vi "Connecting Points.vi"(1 "Boolean":bool, 3 "数组":dbl[][](array[numeric])) -> (0 "输出数组":T1(array[cluster]))   [LabVIEW 2016]
panel:
  out "输出数组 2":dbl[](array[numeric])
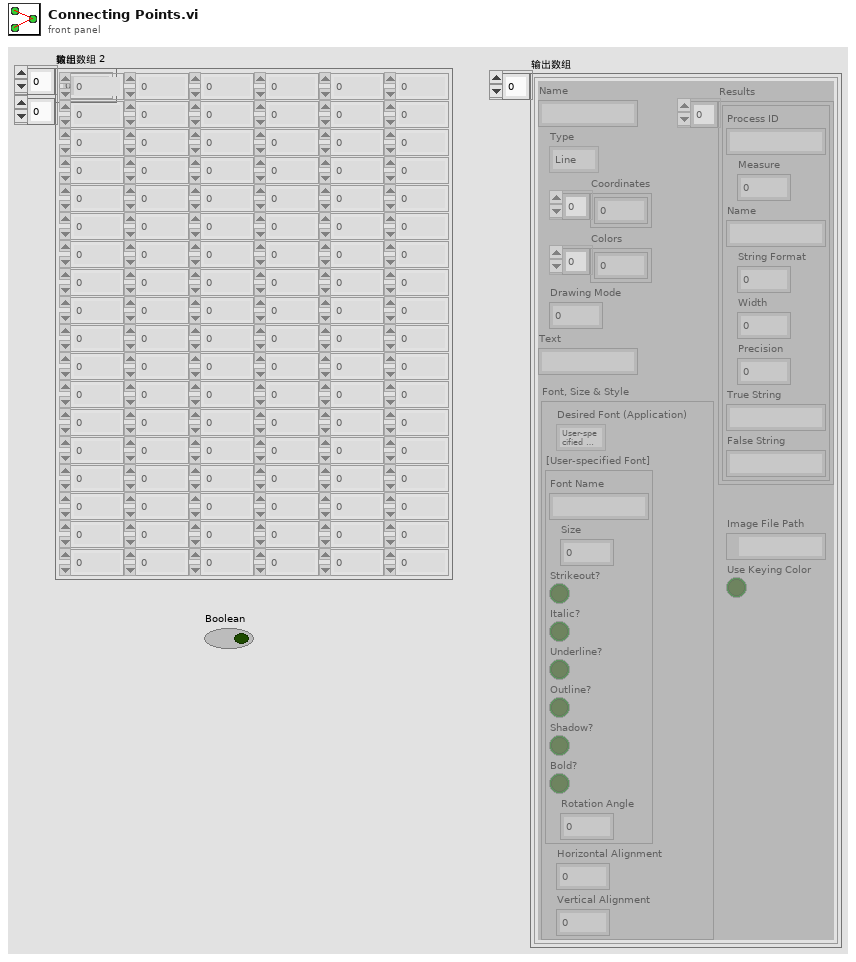
[diagram p1: front panel]
types:
  T1 = cluster{"Name":string, "Type":enum16{"Line", "Broken Line", "Free Hand Line", "Rotated Rectangle", "Oval", "Polygon", "Free Hand", "Bitmap", "Text"}, "Coordinates":i32[], "Colors":u32[], "Drawing Mode":u32, "Text":string, "Results":cluster{"Process ID":string, "Measure":u16, "Name":string, "String Format":u16, "Width":i16, "Precision":i16, "True String":string, "False String":string}[], "Font, Size & Style":cluster{"Desired Font (Application)":enum16{"User-specified Font", "Application Font", "System Font", "Dialog Font"}, "[User-specified Font]":cluster{"Font Name":string, "Size":i16, "Strikeout?":bool, "Italic?":bool, "Underline?":bool, "Outline?":bool, "Shadow?":bool, "Bold?":bool, "Rotation Angle":dbl}, "Horizontal Alignment":i16, "Vertical Alignment":i16}, "Image File Path":path, "Use Keying Color":bool}[]
  T2 = enum16{"Line", "Broken Line", "Free Hand Line", "Rotated Rectangle", "Oval", "Polygon", "Free Hand", "Bitmap", "Text"}
  T3 = cluster{"Name":string, "Type":enum16{"Line", "Broken Line", "Free Hand Line", "Rotated Rectangle", "Oval", "Polygon", "Free Hand", "Bitmap", "Text"}, "Coordinates":i32[], "Colors":u32[], "Drawing Mode":u32, "Text":string, "Results":cluster{"Process ID":string, "Measure":u16, "Name":string, "String Format":u16, "Width":i16, "Precision":i16, "True String":string, "False String":string}[], "Font, Size & Style":cluster{"Desired Font (Application)":enum16{"User-specified Font", "Application Font", "System Font", "Dialog Font"}, "[User-specified Font]":cluster{"Font Name":string, "Size":i16, "Strikeout?":bool, "Italic?":bool, "Underline?":bool, "Outline?":bool, "Shadow?":bool, "Bold?":bool, "Rotation Angle":dbl}, "Horizontal Alignment":i16, "Vertical Alignment":i16}, "Image File Path":path, "Use Keying Color":bool}
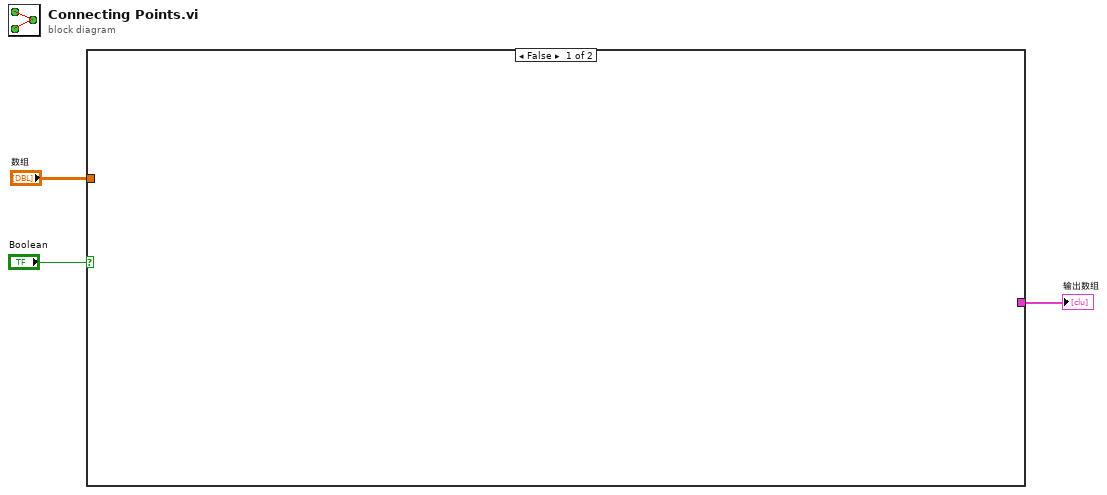
[diagram p0: block diagram]
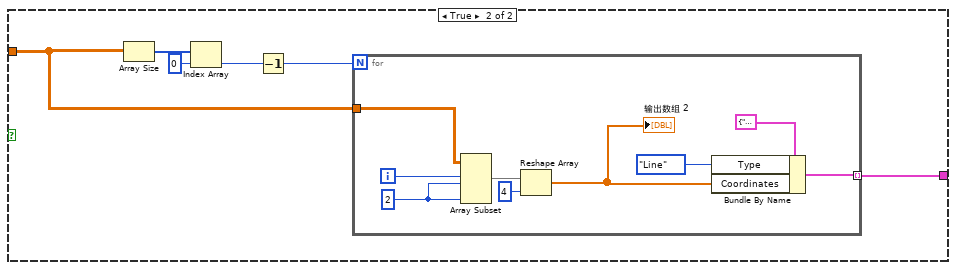
[diagram p2: hidden frame]
diagram:
  n1 = case shown="False" "Boolean" {
    tunnel: [_ w7] -> w3
    tunnel: "数组" -> [_ w6]
    frame False {
    }
    frame True {
      n2 = Array Size(array=w6) -> (size(s)=w8:i32[])
      n3 = Index Array(array=w8, index=0 ("索引")) -> (element=w5:i32)
      n4 = Decrement(x=w5) -> (x-1=w4:i32)
      n5 = for {
        N: w4 -> [_]
        tunnel: [w18] -> w7 mode=indexing
        tunnel: w6 -> [w15]
        i -> [w14]
        w13 = 2 ("长度")
        n6 = Array Subset(array=w15, index (row)=w14, length (row)=w13, length (col)=w13) -> (w12:dbl[][])  [unwired: 1 in]
        n7 = Reshape Array(w12, 4 ("维数大小")) -> (w11:dbl[])
        "输出数组 2" <- w11
        n8 = Bundle By Name(cluster=T3 {"Name"="Line 1", "Type"=enum."Line", "Coordinates"=[606, 1151, 1346, 834], "Colors"=[16711680], "Drawing Mode"=0, "Text"="Your Text", "Results"=[], "Font, Size & Style"={"Desired Font (Application)"=enum."System Font", "[User-specified Font]"={"Font Name"="Tahoma", "Size"=13, "Strikeout?"=FALSE, "Italic?"=FALSE, "Underline?"=FALSE, "Outline?"=FALSE, "Shadow?"=FALSE, "Bold?"=FALSE, "Rotation Angle"=0.0}, "Horizontal Alignment"=0, "Vertical Alignment"=0}, "Image File Path"=path "", "Use Keying Color"=FALSE} ("Overlay"), "Type"=T2."Line", "Coordinates"=w11) -> (w18:T3)
      }
    }
  }
  "输出数组" <- w3
